vi "IoT_VIs.vi"() -> ()   [LabVIEW 2019]
panel:
  out "resulting string":string
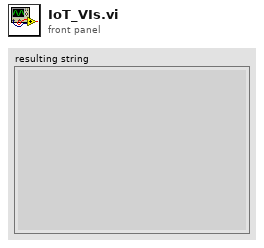
[diagram p1: front panel]
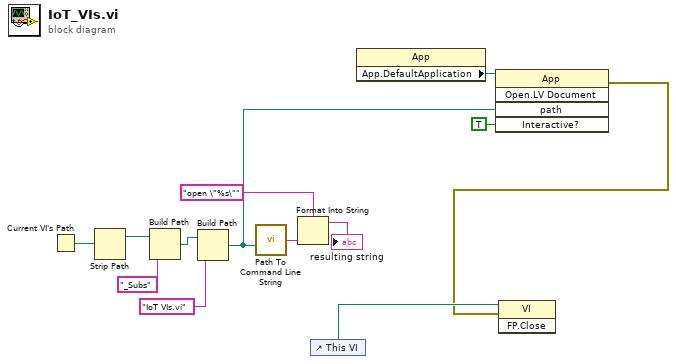
[diagram p0: block diagram]
diagram:
  n1 = Current VI's Path() -> (path=w13:path)
  n2 = Strip Path(path=w13) -> (stripped path=w12:path)  [unwired: 1 out]
  n3 = Build Path(base path=w12, name or relative path="_Subs") -> (appended path=w11:path)
  n4 = Build Path(base path=w11, name or relative path="IoT VIs.vi") -> (appended path=w2:path)
  n5 = call <vilib>:"Path To Command Line String.vi"("path"=w2) -> ("string"=w8:string)
  n6 = Format Into String(format string="open \"%s\"" ("command line"), w8) -> (resulting string=→"resulting string":string)  [unwired: 2 in, 1 out]
  n7 = control-ref of="This VI"() -> (w5:refnum<vi>)
  n8 = property class="App"() -> ("App.DefaultApplication"=w4:refnum<vi>)  [unwired: 2 in, 2 out]
  n9 = invoke class="App" method="Open.LV Document"(reference=w4, "path"=w2, "Interactive?"=TRUE) -> (error out=w1:errorcluster)  [unwired: 2 in, 4 out]
  n10 = invoke class="VI" method="FP.Close"(reference=w5, error in=w1) -> ()  [unwired: 1 in, 3 out]
